vi "Helper SubVI - Get Single-level Detail Coefficients.vi"(9 "index of Lengths":i32, 10 "Lengths":i32[](array[numeric]), 11 "DWT":dbl[](array[numeric])) -> (1 "Lengths out":i32[](array[numeric]), 2 "DWT 2":dbl[](array[numeric]), 3 "Coeffs":dbl[](array[numeric]))   [LabVIEW 2023]
doc: "Gets the single-level detail coefficients."
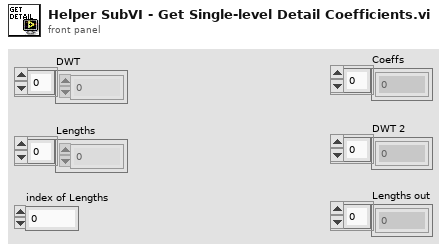
[diagram p1: front panel]
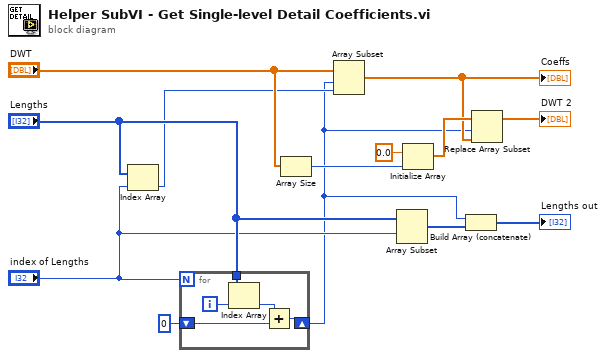
[diagram p0: block diagram]
diagram:
  n1 = Index Array(array="Lengths", index="index of Lengths") -> (element=w2:i32)
  n2 = for {
    N: "index of Lengths" -> [_]
    shift-right: [w15] -> w1
    shift-left: 0 -> [w16]
    tunnel: "Lengths" -> [w18]
    i -> [w14]
    n3 = Index Array(array=w18, index=w14) -> (element=w17:i32)
    n4 = Add(x=w17, y=w16) -> (x+y=w15:i32)
  }
  n5 = Array Size(array="DWT") -> (size(s)=w7:i32)
  n6 = Array Subset(array="DWT", index=w1, length=w2) -> (w5:dbl[])
  "Coeffs" <- w5
  n7 = Array Subset(array="Lengths", index="index of Lengths") -> (w11:i32[])  [unwired: 1 in]
  n8 = Initialize Array(0.0 ("element"), w7) -> (w6:dbl[])
  n9 = Build Array (concatenate)(w1, w11) -> (→"Lengths out":i32[])
  n10 = Replace Array Subset(array=w6, new element=w5, index=w1) -> (→"DWT 2":dbl[])
